vi "deploy next logic.vi"(8 "error in (no error)":errorcluster, 10 "Rename":refnum<vi>, 11 "TabControl in":refnum<vi>) -> (0 "error out":errorcluster, 1 "Tab Control":T4, 2 "Button state":T3, 3 "Execution state":T2, 4 "UI Screen out":T1)   [LabVIEW 2013]
uses:
  types/TabStateType.ctl
  types/ButtonStateType.ctl
  types/ExecutionStateType.ctl
  types/UserStateType.ctl
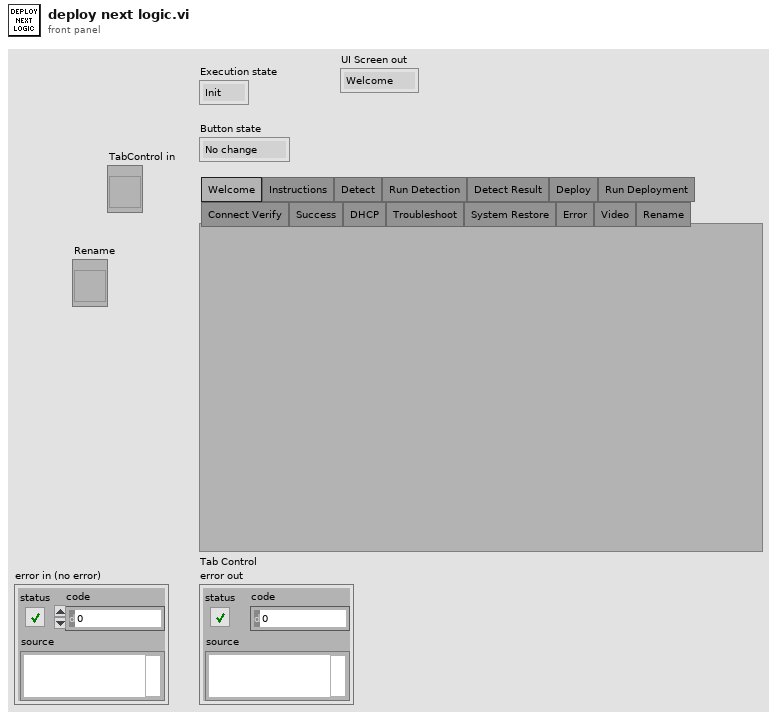
[diagram p1: front panel]
types:
  T1 = typedef "UserStateType.ctl" = enum16{"Welcome", "Instructions", "Detect", "Deploy", "Success"}
  T2 = typedef "ExecutionStateType.ctl" = enum16{"Init", "Welcome", "Idle", "Detect", "Run Detection", "Detect Fail", "Detect One", "Detect Mult", "Deploy", "DHCP", "Static IP", "Run Deployment", "Connect Verify", "Exit", "Video Wait", "Success", "Troubleshoot", "Troubleshoot 2", "RenameDNS"}
  T3 = typedef "ButtonStateType.ctl" = enum16{"No change", "No Next", "No Prev", "All Disabled", "All Enabled", "Exit Only"}
  T4 = typedef "TabStateType.ctl" = enum32{"Welcome", "Instructions", "Detect", "Run Detection", "Detect Result", "Deploy", "Run Deployment", "Connect Verify", "Success", "DHCP", "Troubleshoot", "System Restore", "Error", "Video", "Rename"}
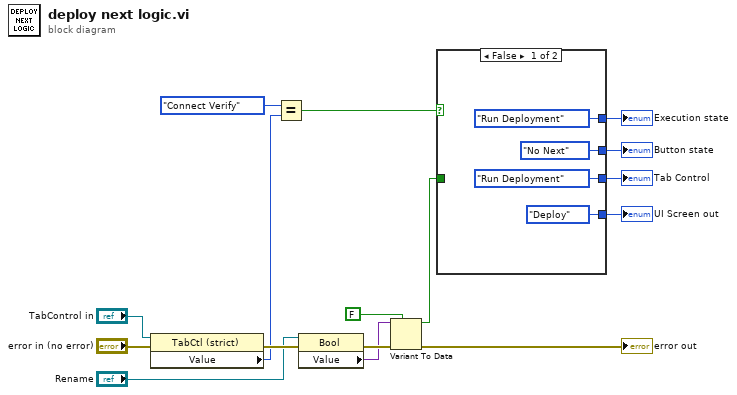
[diagram p0: block diagram]
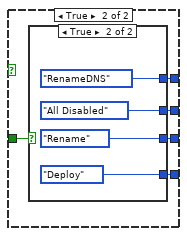
[diagram p2: hidden frame]
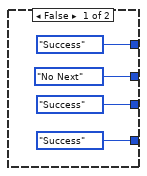
[diagram p3: hidden frame]
diagram:
  n1 = property class="TabCtl (strict)"(reference="TabControl in", error in="error in (no error)") -> (error out=w9:errorcluster, "Value"=w3:T4)  [unwired: 1 out]
  n2 = Equal?(x=TabStateType."Connect Verify" ("y"), y=w3) -> (x = y?=w13:bool)
  n3 = property class="Bool"(reference="Rename", error in=w9) -> (error out=w7:errorcluster, "Value"=w6:variant)  [unwired: 1 out]
  n4 = Variant To Data(error in=w7, type=FALSE, Variant=w6) -> (data=w4:bool, error out=→"error out":errorcluster)
  n5 = case shown="False" w13 {
    tunnel: [ExecutionStateType."Run Deployment" ("Enum") w24] -> w14
    tunnel: [ButtonStateType."No Next" ("Enum") w23] -> w15
    tunnel: [TabStateType."Run Deployment" ("Tab Control") w22] -> w16
    tunnel: w4 -> [_ w25]
    tunnel: [UserStateType."Deploy" ("UI Screen in out") w21] -> w1
    frame False {
    }
    frame True {
      n6 = case shown="True" w25 {
        tunnel: [ExecutionStateType."Success" ("Enum") ExecutionStateType."RenameDNS" ("Enum")] -> w24
        tunnel: [ButtonStateType."No Next" ("Enum") ButtonStateType."All Disabled" ("Enum")] -> w23
        tunnel: [TabStateType."Success" ("Tab Control") TabStateType."Rename" ("Tab Control")] -> w22
        tunnel: [UserStateType."Success" ("UI Screen in out") UserStateType."Deploy" ("UI Screen in out")] -> w21
        frame False {
        }
        frame True {
        }
      }
    }
  }
  "Tab Control" <- w16
  "Button state" <- w15
  "Execution state" <- w14
  "UI Screen out" <- w1
